vi "WriteConfigSettings.vi"(6 "# columns after Trig (0-128)":u16=120, 7 "QDC High threshold":u16=1, 8 "QDC Low threshold":u16=1, 9 "TDC bin width (ns)":dbl format="%#_13g", 10 "TDC Low Range threshold (bins)":u16=1, 11 "ref in":T1 format="%.0x") -> (0 "error out":errorcluster)   [LabVIEW 2014]
uses:
  <vilib>/addons/h5labview2/base/hid_t.ctl
  <vilib>/addons/h5labview2/base/lib_path.vi
  <vilib>/addons/h5labview2/base/H5Equery.vi
  <vilib>/addons/h5labview2/dataset/H5Dwrite.llb/H5Dwrite.xnode
  <vilib>/addons/h5labview2/group/H5G.lvlib
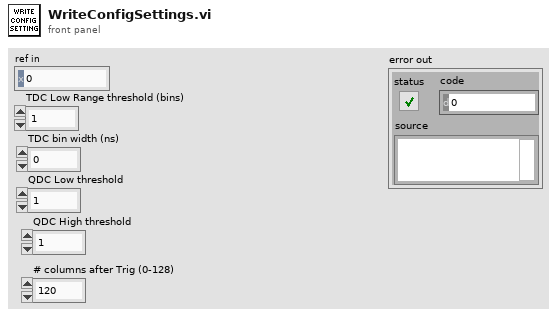
[diagram p1: front panel]
types:
  T1 = typedef "hid_t.ctl" = i32
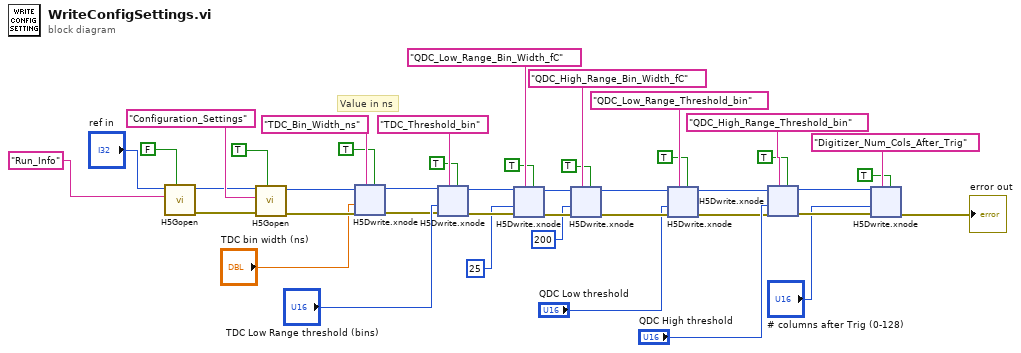
[diagram p0: block diagram]
diagram:
  # "Value in ns"
  n1 = call <vilib>:"H5Gopen.vi"("create? (F)"=FALSE, "name"="Run_Info", "ref in"="ref in") -> ("error out"=w38:errorcluster, "group out"=w39:T1)  [unwired: 7 in]
  n2 = call <vilib>:"H5Gopen.vi"("create? (F)"=TRUE, "error in (no error)"=w38, "name"="Configuration_Settings", "ref in"=w39) -> ("error out"=w35:errorcluster, "group out"=w36:T1)  [unwired: 6 in]
  n3 = xnode "H5Dwrite.xnode"("replace? (F)"=TRUE, "dataset name"="TDC_Bin_Width_ns", "error in (no error)"=w35, "data"="TDC bin width (ns)", "ref in"=w36) -> ("error out"=w27:errorcluster, "ref out"=w31:i32)  [unwired: 2 in, 1 out]
  n4 = xnode "H5Dwrite.xnode"("replace? (F)"=TRUE, "dataset name"="TDC_Threshold_bin", "error in (no error)"=w27, "data"="TDC Low Range threshold (bins)", "ref in"=w31) -> ("error out"=w23:errorcluster, "ref out"=w24:i32)  [unwired: 2 in, 1 out]
  n5 = xnode "H5Dwrite.xnode"("replace? (F)"=TRUE, "dataset name"="QDC_Low_Range_Bin_Width_fC", "error in (no error)"=w23, "data"=u8 25, "ref in"=w24) -> ("error out"=w19:errorcluster, "ref out"=w18:i32)  [unwired: 2 in, 1 out]
  n6 = xnode "H5Dwrite.xnode"("replace? (F)"=TRUE, "dataset name"="QDC_High_Range_Bin_Width_fC", "error in (no error)"=w19, "data"=u8 200, "ref in"=w18) -> ("error out"=w13:errorcluster, "ref out"=w14:i32)  [unwired: 2 in, 1 out]
  n7 = xnode "H5Dwrite.xnode"("replace? (F)"=TRUE, "dataset name"="QDC_Low_Range_Threshold_bin", "error in (no error)"=w13, "data"="QDC Low threshold", "ref in"=w14) -> ("error out"=w7:errorcluster, "ref out"=w8:i32)  [unwired: 2 in, 1 out]
  n8 = xnode "H5Dwrite.xnode"("replace? (F)"=TRUE, "dataset name"="QDC_High_Range_Threshold_bin", "error in (no error)"=w7, "data"="QDC High threshold", "ref in"=w8) -> ("error out"=w6:errorcluster, "ref out"=w5:i32)  [unwired: 2 in, 1 out]
  n9 = xnode "H5Dwrite.xnode"("replace? (F)"=TRUE, "dataset name"="Digitizer_Num_Cols_After_Trig", "error in (no error)"=w6, "data"="# columns after Trig (0-128)", "ref in"=w5) -> ("error out"=→"error out":errorcluster)  [unwired: 2 in, 2 out]
